vi "set_number_of_channels.vi"(8 "error in (no error)":errorcluster, 10 "number of channels":i32, 11 "GenericImageAssembler.lvclass in":refnum<class "GenericImageAssembler.lvclass">) -> (0 "error out":errorcluster, 3 "GenericImageAssembler.lvclass out":refnum<class "GenericImageAssembler.lvclass">)   [LabVIEW 2010, in "GenericImageAssembler.lvclass"]
uses:
  GenericImageAssembler.lvclass
  GenericImageAssembler.lvclass/GenericImageAssembler.ctl
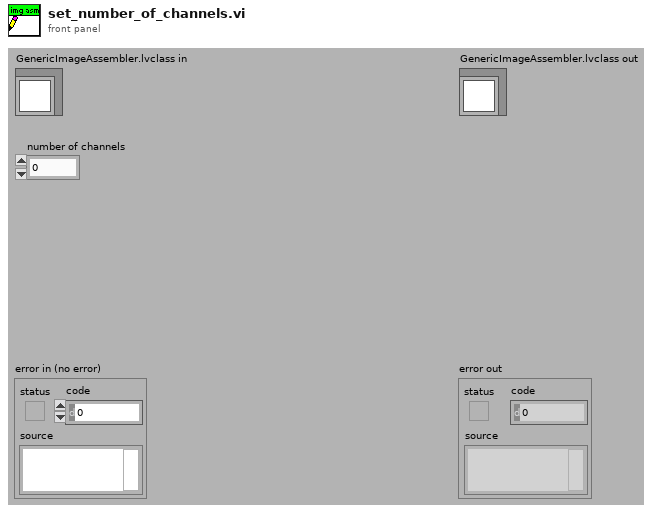
[diagram p1: front panel]
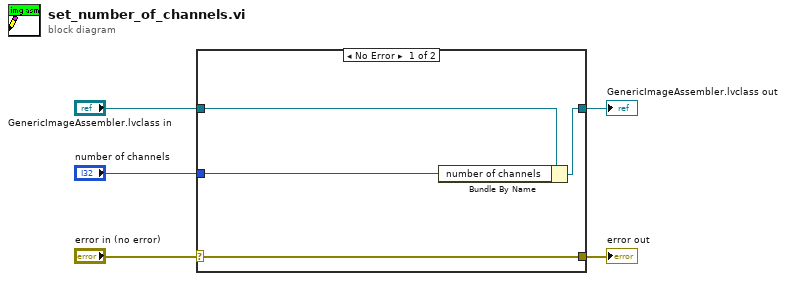
[diagram p0: block diagram]
diagram:
  n1 = case shown="No Error" "error in (no error)" {
    selector: "error in (no error)" -> [w9 w10]
    tunnel: [w9 w10] -> w4
    tunnel: [w7 w11] -> w2
    tunnel: "GenericImageAssembler.lvclass in" -> [w8 w11]
    tunnel: "number of channels" -> [w6 _]
    frame No Error {
      n2 = Bundle By Name(cluster=w8, "number of channels"=w6) -> (w7:refnum<class "GenericImageAssembler.lvclass">)
    }
    frame Error {
    }
  }
  "error out" <- w4
  "GenericImageAssembler.lvclass out" <- w2
